vi "Decode.vi"(8 "error in (no error)":errorcluster, 10 "Message":string, 11 "Actuator in":refnum<class "Actuator.lvclass">) -> (0 "error out":errorcluster, 3 "Actuator out":refnum<class "Actuator.lvclass">)   [LabVIEW 2021, in "Actuator.lvclass"]
uses:
  Actuator.lvclass
panel:
  out "remaining string":string
  out "PWM":i32
  out "On":i32
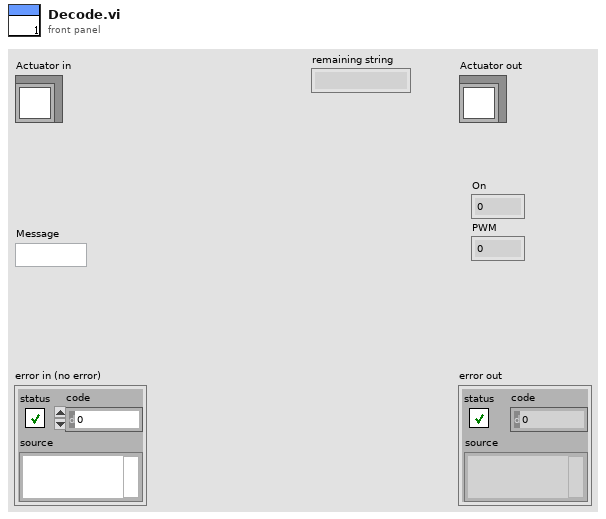
[diagram p1: front panel]
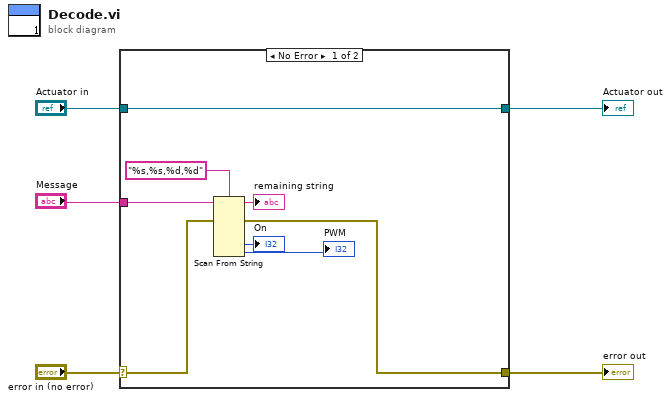
[diagram p0: block diagram]
diagram:
  n1 = case shown="No Error" "error in (no error)" {
    selector: "error in (no error)" -> [w7 w15]
    tunnel: [w6 w15] -> w4
    tunnel: [w13 w14] -> w2
    tunnel: "Actuator in" -> [w13 w14]
    tunnel: "Message" -> [w12 _]
    frame No Error {
      n2 = Scan From String(format string="%s,%s,%d,%d", input string=w12, error in=w7) -> (remaining string=→"remaining string":string, error out=w6:errorcluster, output 3=→"On":i32, output 4=→"PWM":i32)  [unwired: 7 in, 1 out]
    }
    frame Error {
    }
  }
  "error out" <- w4
  "Actuator out" <- w2
